vi "Tx.vi"(8 "error in (no error)":errorcluster, 10 "Transfer Group in":refnum<class "Transfer Group.lvclass">, 11 "Transceiver Thread in":refnum<class "Transceiver Thread.lvclass">) -> (0 "error out":errorcluster, 2 "Transfer Group out":refnum<class "Transfer Group.lvclass">, 3 "Transceiver Thread out":refnum<class "Transceiver Thread.lvclass">)   [LabVIEW 2019, in "DSF Core.lvlib" / "Transceiver Thread.lvclass"]
uses:
  Transceiver Thread.lvclass
  Transfer Group/Transfer Group.lvclass
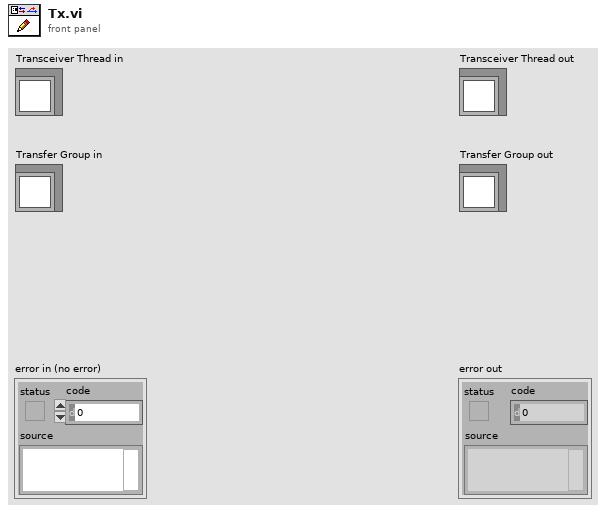
[diagram p1: front panel]
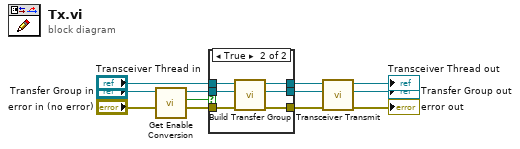
[diagram p0: block diagram]
diagram:
  n1 = call "Get Enable Conversion.vi"("Transfer Group in"="Transfer Group in") -> ("enable conversion"=w1:bool, "Transfer Group out"=w2:refnum<class "Transfer Group.lvclass">)  [unwired: 9 in]
  n2 = case shown="True" w1 {
    tunnel: "Transceiver Thread in" -> [w13 w20]
    tunnel: "error in (no error)" -> [w12 w19]
    tunnel: [w13 w18] -> w6
    tunnel: [w14 w17] -> w5
    tunnel: [w12 w16] -> w4
    tunnel: w2 -> [w14 w15]
    frame False {
    }
    frame True {
      n3 = call "Build Transfer Group.vi"("error in (no error)"=w19, "Transfer Group in"=w15, "Plugin Thread in"=w20) -> ("error out"=w16:errorcluster, "Transfer Group out"=w17:refnum<class "Transfer Group.lvclass">, "Plugin Thread out"=w18:refnum<class "Transceiver Thread.lvclass">)  [unwired: 6 in]
    }
  }
  n4 = call "Transceiver Transmit.vi"("error in (no error)"=w4, "Transfer Group in"=w5, "Transceiver Thread in"=w6) -> ("error out"=→"error out":errorcluster, "Transfer Group out"=→"Transfer Group out":refnum<class "Transfer Group.lvclass">, "Transceiver Thread out"=→"Transceiver Thread out":refnum<class "Transceiver Thread.lvclass">)  [unwired: 6 in]
